vi "fgv_joystick_config.vi"(7 "cmd":T3, 8 "error in":errorcluster, 11 "Joystick cfg 2":T1={"steer limit"={"scale"=10.0, "offset"=42.0}, "speed limit"={"min"=10.0, "max"=42.0}, "Axis"={"man"=0.0, "auto"=0.0, "angular"=enum."X axis", "linear"=enum."Z rotation", "linear inv"=FALSE, "ang inv"=FALSE}} {"speed limit"."max" min=0.0 max=254.0 step=1.0}) -> (0 "error out":errorcluster, 3 "Joystick cfg 3":T1={"steer limit"={"scale"=10.0, "offset"=42.0}, "speed limit"={"min"=10.0, "max"=42.0}, "Axis"={"man"=0.0, "auto"=0.0, "angular"=enum."X axis", "linear"=enum."Z rotation", "linear inv"=FALSE, "ang inv"=FALSE}} {"speed limit"."max" min=0.0 max=254.0 step=1.0})   [LabVIEW 2021]
uses:
  Ctrl/cmd_common.ctl
  Ctrl/joystick cfg.ctl
  Ctrl/joy-axis.ctl
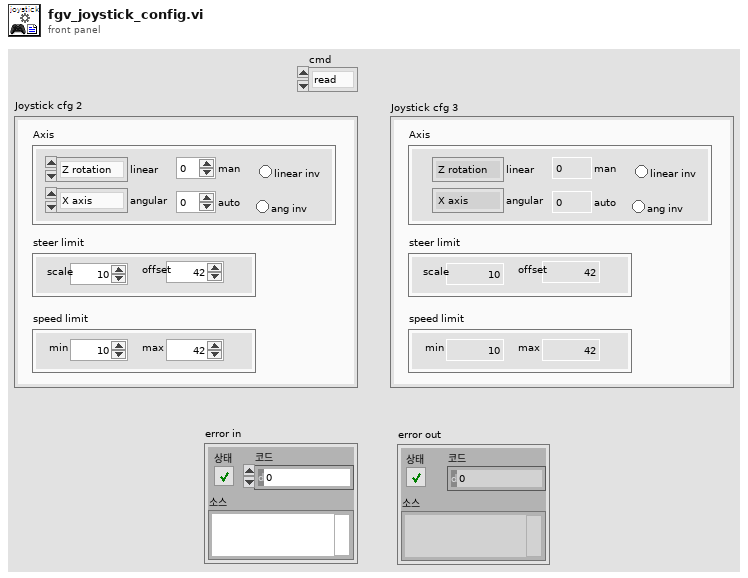
[diagram p1: front panel]
types:
  T1 = typedef "joystick cfg.ctl" = cluster{"steer limit":cluster{"scale":dbl, "offset":dbl}, "speed limit":cluster{"min":dbl, "max":dbl}, "Axis":cluster{"man":dbl, "auto":dbl, "angular":T2, "linear":T2, "linear inv":bool, "ang inv":bool}}
  T2 = typedef "joy-axis.ctl" = enum16{"X axis", "Y axis", "Z axis", "X rotation", "Y rotation", "Z rotation", "U axis", "V axis"}
  T3 = typedef "cmd_common.ctl" = enum16{"read", "write"}
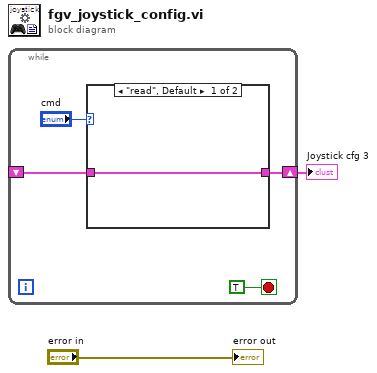
[diagram p0: block diagram]
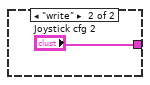
[diagram p2: hidden frame]
diagram:
  n1 = while {
    shift-right: [w4] -> w1
    shift-left: _ -> [w3]
    stop <- TRUE stop-if-true
    n2 = case shown="\"read\", Default" "cmd" {
      tunnel: [w7 "Joystick cfg 2"] -> w4
      tunnel: w3 -> [w7 _]
      frame "read", Default {
      }
      frame "write" {
      }
    }
  }
  "Joystick cfg 3" <- w1
  "error out" <- "error in"
